vi "Launch View.vi"(8 "error in (no error)":errorcluster, 11 "base view in":refnum<class "base view.lvclass">) -> (0 "error out":errorcluster, 3 "base view out":refnum<class "base view.lvclass">)   [LabVIEW 2022 SP3, in "base view.lvclass"]
uses:
  base view.lvclass
  Run View.vi
  Accessors/Read Events.vi
  Accessors/Write Event Registration Refnum.vi
  Accessors/Write Wrapped View Refnum.vi
  Accessors/Read View Refnum.vi
  base view.lvclass/base view.ctl
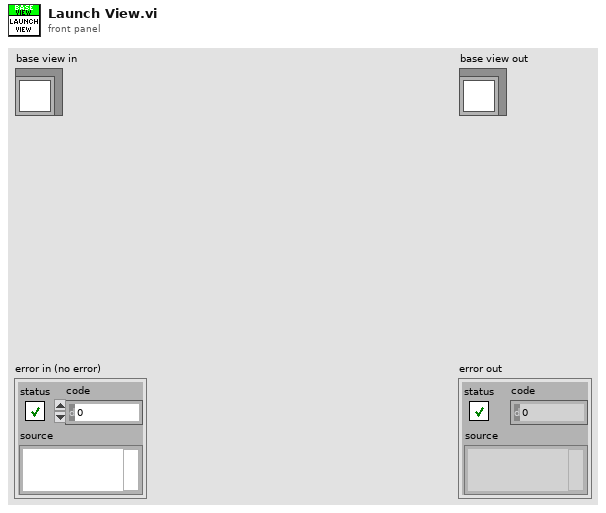
[diagram p1: front panel]
types:
  T1 = typedef "base view.lvclass/Events.ctl" = cluster{"Open":refnum<user-event>, "Close":refnum<user-event>, "Hide":refnum<user-event>}
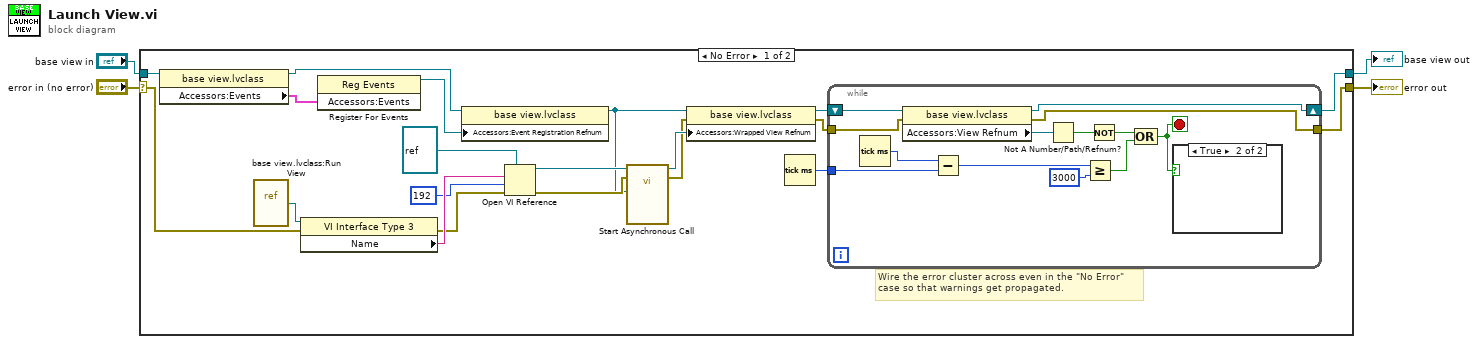
[diagram p0: block diagram]
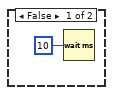
[diagram p2: hidden frame]
diagram:
  n1 = case shown="No Error" "error in (no error)" {
    selector: "error in (no error)" -> [w19 w40]
    tunnel: [w9 w40] -> w3
    tunnel: [w12 w39] -> w1
    tunnel: "base view in" -> [w16 w39]
    frame No Error {
      # "Wire the error cluster across even in the \"No Error\"\ncase so that warnings get propagated."
      n2 = property class="base view.lvclass"(reference=w16) -> (reference out=w8:refnum<class "base view.lvclass">, "Accessors:Events"=w7:T1)  [unwired: 1 in, 1 out]
      n3 = vi-ref "base view.lvclass:Run View.vi"() -> (w24:refnum<vi>)
      n4 = property class="VI Interface Type 3"(reference=w24, error in=w19) -> (error out=w18:errorcluster, "Name"=w23:string)  [unwired: 1 out]
      n5 = register-events(w7) -> (reference out=w5:refnum<event-registration>)  [unwired: 2 in, 1 out]
      n6 = property class="base view.lvclass"(reference=w8, "Accessors:Event Registration Refnum"=w5) -> (reference out=w6:refnum<class "base view.lvclass">)  [unwired: 1 in, 1 out]
      n7 = Open VI Reference(type specifier VI Refnum (for type only)=refnum<vi> refnum, vi path=w23, options=192, error in (no error)=w18) -> (vi reference=w21:refnum<vi>, error out=w17:errorcluster)  [unwired: 2 in]
      n8 = call-by-ref "Start Asynchronous Call"(reference=w21, error in=w17, "base view in"=w6) -> (reference out=w15:refnum<vi>, error out=w11:errorcluster)  [unwired: 9 in, 2 out]
      n9 = property class="base view.lvclass"(reference=w6, error in=w11, "Accessors:Wrapped View Refnum"=w15) -> (reference out=w13:refnum<class "base view.lvclass">, error out=w10:errorcluster)
      n10 = Tick Count (ms)() -> (millisecond timer value=w14:u32)
      n11 = while {
        tunnel: w14 -> [w36]
        shift-right: [w28] -> w12
        shift-left: w13 -> [w33]
        tunnel: w10 -> [w26]
        tunnel: [w25] -> w9
        stop <- w27 stop-if-true
        n12 = Tick Count (ms)() -> (millisecond timer value=w37:u32)
        n13 = property class="base view.lvclass"(reference=w33, error in=w26) -> (reference out=w28:refnum<class "base view.lvclass">, error out=w25:errorcluster, "Accessors:View Refnum"=w32:refnum<vi>)
        n14 = Subtract(x=w37, y=w36) -> (x-y=w35:u32)
        n15 = Not A Number/Path/Refnum?(number/path/refnum=w32) -> (NaN/Path/Refnum?=w31:bool)
        n16 = Greater Or Equal?(x=w35, y=u32 3000) -> (x >= y?=w29:bool)
        n17 = Not(x=w31) -> (.not. x?=w30:bool)
        n18 = Compound Arithmetic op=OR(w30, w29) -> (w27:bool)
        n19 = case shown="True" w27 {
          frame False {
            n20 = Wait (ms)(milliseconds to wait=u32 10) -> ()  [unwired: 1 out]
          }
          frame True {
          }
        }
      }
    }
    frame Error {
    }
  }
  "error out" <- w3
  "base view out" <- w1
